vi "Generate Digital Codes.vi"(6 "Input Code Bit":enum16{"16-Bit", "12-Bit"}(ring), 7 "Command":enum16{"Read", "Write"}(ring)=enum."Write", 9 "Address":u8=128 format="%.0x", 10 "End code":u16=3968, 11 "Start code":u16=32) -> (3 "Digital commands":i16[](array[numeric]), 4 "Command size":u16, 5 "Number of commands":u16)   [LabVIEW 2021]
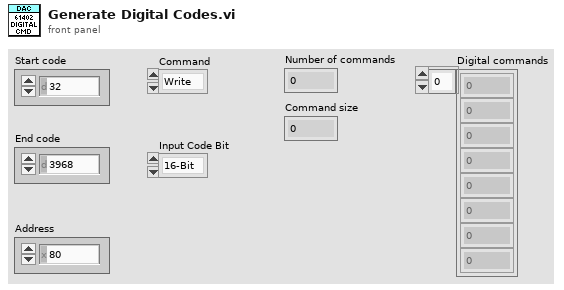
[diagram p1: front panel]
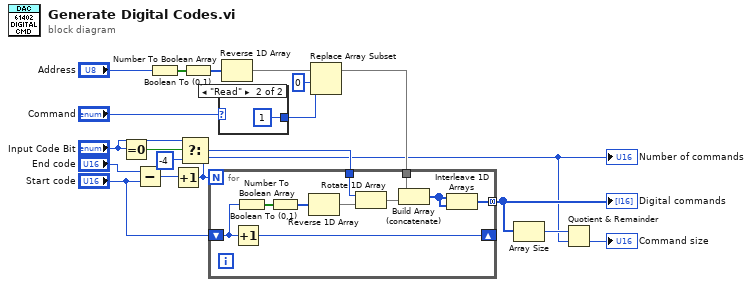
[diagram p0: block diagram]
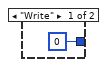
[diagram p2: hidden frame]
diagram:
  n1 = Equal To 0?(x="Input Code Bit") -> (x = 0?=w8:bool)
  n2 = Subtract(x="End code", y="Start code") -> (x-y=w18:u16)
  n3 = Number To Boolean Array(number="Address") -> (Boolean array=w15:bool[])
  n4 = Increment(x=w18) -> (x+1=w2:u16)
  "Number of commands" <- w2
  n5 = Select(t="Input Code Bit", s=w8, f=-4 ("n")) -> (s? t:f=w5:i32)
  n6 = Boolean To (0,1)(Boolean=w15) -> (0, 1=w16:i16[])
  n7 = case shown="\"Read\"" "Command" {
    tunnel: [i16 0 i16 1] -> w11
    frame "Write" {
    }
    frame "Read" {
    }
  }
  n8 = Reverse 1D Array(array=w16) -> (reversed array=w12:i16[])
  n9 = Replace Array Subset(array=w12, new element=w11, index=0) -> (w9:i16[])
  n10 = for {
    N: w2 -> [_]
    shift-right: [w30] -> _
    shift-left: "Start code" -> [w28]
    tunnel: [w27] -> w4 mode=concatenating
    tunnel: w9 -> [w26]
    tunnel: w5 -> [w22]
    n11 = Increment(x=w28) -> (x+1=w30:u16)
    n12 = Number To Boolean Array(number=w28) -> (Boolean array=w31:bool[])
    n13 = Boolean To (0,1)(Boolean=w31) -> (0, 1=w29:i16[])
    n14 = Reverse 1D Array(array=w29) -> (reversed array=w24:i16[])
    n15 = Rotate 1D Array(1:w24, 2:w22) -> (0:w23:i16[])
    n16 = Build Array (concatenate)(w26, w23) -> (w25:i16[])
    n17 = Interleave 1D Arrays(w25, w25) -> (w27:i16[])
  }
  "Digital commands" <- w4
  n18 = Array Size(array=w4) -> (size(s)=w3:i32)
  n19 = Quotient & Remainder(x=w3, y=w2) -> (floor(x/y)=→"Command size":i32)  [unwired: 1 out]
